vi "Stack-visualise.vi"() -> ()   [LabVIEW 2018]
uses:
  <vilib>/vision/NI_Vision_Development_Module.lvlib
panel:
  out "Numeric":i32
  in  "Stop":bool
  in  "Slide":dbl(slide) scale=0.0..800.0
  out "Image":T1(plugin-control)
  out "filenames":string[](array[string])
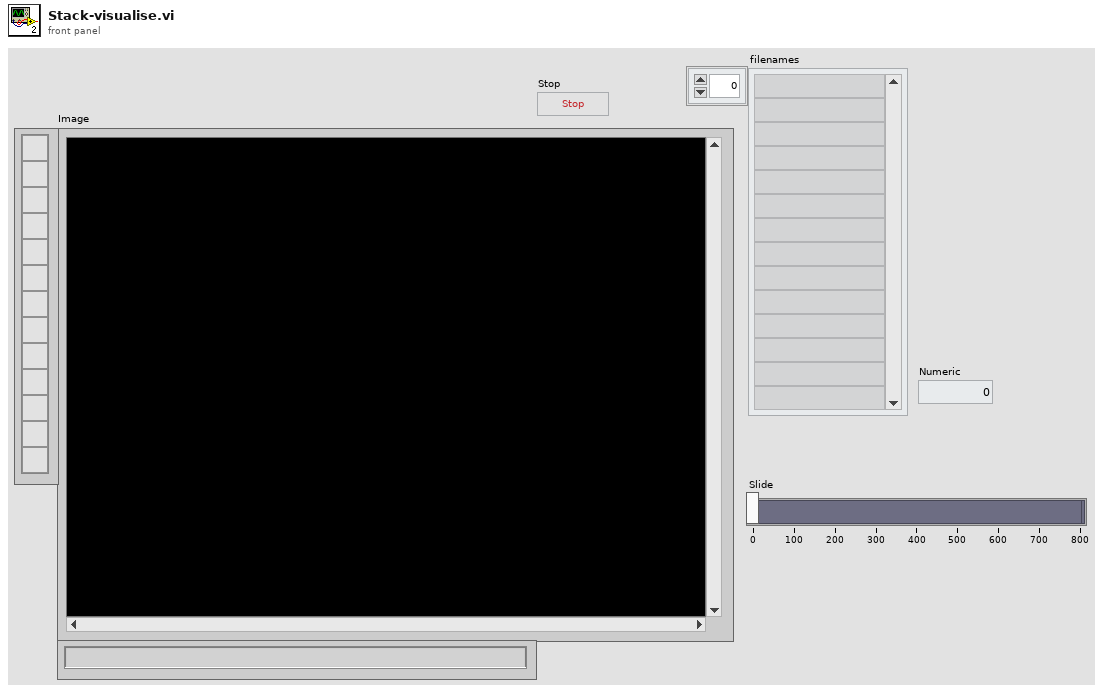
[diagram p1: front panel]
types:
  T1 = typedef "IMAQ Image.ctl" = refnum<image>
  T2 = cluster{"Global Rectangle":i32[], "Contours":cluster{"Contour Type":u32, "ROI Type":u32, "Points":i32[]}[]}
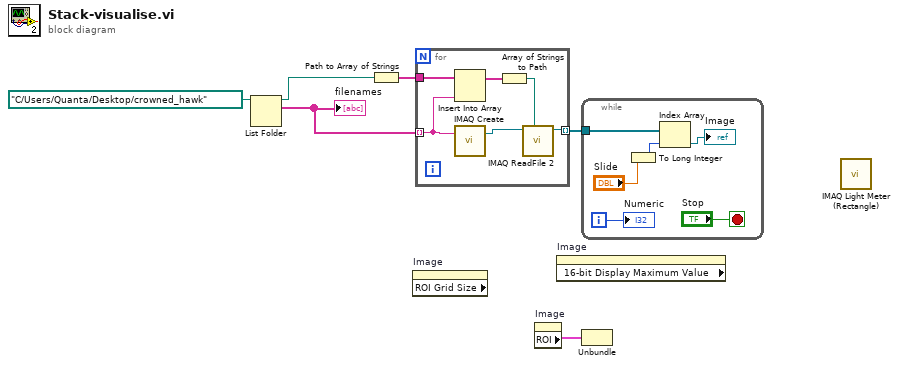
[diagram p0: block diagram]
diagram:
  n1 = List Folder(path=path "C:/Users/Quanta/Desktop/crowned_hawk") -> (path out=w5:path, filenames=w3:string[])  [unwired: 3 in, 2 out]
  "filenames" <- w3
  n2 = Path to Array of Strings(0:w5) -> (2:w4:string[])  [unwired: 1 out]
  n3 = property on="Image" class="ImageControl" props=["ROI Grid Size"]() -> ()  [unwired: 2 in, 3 out]
  n4 = for {
    tunnel: w3 -> [w9] mode=indexing
    tunnel: [w11] -> w2 mode=indexing
    tunnel: w4 -> [w10]
    n5 = Insert Into Array(array=w10, new element=w9) -> (w8:string[])  [unwired: 1 in]
    n6 = call "IMAQ Create"("Image Name"=w9) -> ("New Image"=w12:T1)  [unwired: 4 in, 1 out]
    n7 = Array of Strings to Path(0:w8) -> (2:w7:path)  [unwired: 1 in]
    n8 = call "IMAQ ReadFile 2"("File Path"=w7, "Image"=w12) -> ("Image Out"=w11:T1)  [unwired: 5 in, 4 out]
  }
  n9 = property on="Image" class="ImageControl"() -> ("ROI"=w1:T2)  [unwired: 2 in, 2 out]
  n10 = property on="Image" class="ImageControl" props=["16-bit Display Maximum Value"]() -> ()  [unwired: 2 in, 3 out]
  n11 = while {
    tunnel: w2 -> [w18]
    i -> [w13]
    stop <- "Stop" stop-if-true
    n12 = To Long Integer(number="Slide") -> (32bit integer=w15:i32)
    n13 = Index Array(array=w18, index=w15) -> (element=→"Image":T1)
    "Numeric" <- w13
  }
  n14 = Unbundle(w1) -> ()  [unwired: 2 out]
  n15 = call "IMAQ Light Meter (Rectangle)"() -> ()  [unwired: 7 in, 5 out]
